vi "Convert Waveform to DDT.vi"() -> ()   [LabVIEW 2011]
doc: "This example shows how to use the Convert to DDT function. Specifically, this example converts the Waveform data type to the Dynamic Data Type, but the Convert to DDT function can also be used to convert 1D or 2D Arrays of doubles and a 1D array of Waveform data. \n\nThe graph plots the multitone wave and the filtered wave. The two signals are combined using the Merge Signals function and have separate Y-axis.\n\nThis example uses the following Express VIs: Convert to DDT and Filter."
uses:
  Instance           2 31Saved   Convert Waveform to DDT .vi
  Instance           3 31Saved   Convert Waveform to DDT .vi
  <vilib>/measure/NI_MAPro.lvlib
panel:
  out "Waveform Graph":dynamicdata(graph)
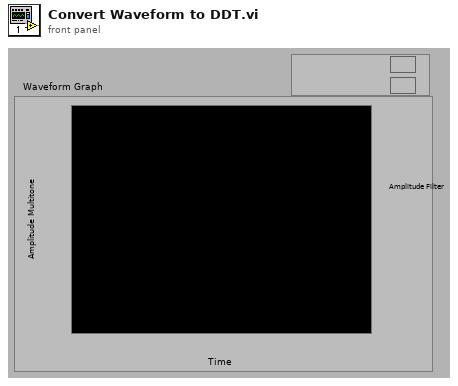
[diagram p1: front panel]
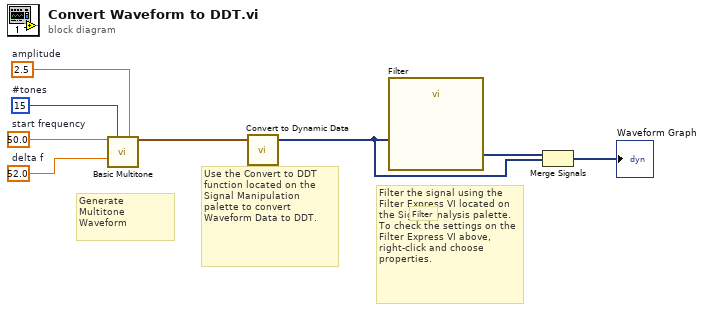
[diagram p0: block diagram]
diagram:
  w5 = 52.0  # delta f
  w6 = 50.0  # start frequency
  w7 = 2.5  # amplitude
  w8 = 15  # #tones
  # "Filter the signal using the Filter Express VI located on the Signal Analysis palette.  To check the settings on the Filter Express VI above, right-click and choose properties."
  # "Use the Convert to DDT function located on the Signal Manipulation palette to convert Waveform Data to DDT."
  # "Filter"
  # "Generate Multitone Waveform"
  n1 = call <vilib>:"Basic Multitone.vi"("start frequency"=w6, "#tones"=w8, "amplitude"=w7, "delta frequency"=w5) -> ("signal out"=w3:waveform(dbl))  [unwired: 6 in, 5 out]
  n2 = call "Convert to Dynamic Data"("Waveform"=w3) -> ("Dynamic Data Type"=w2:dynamicdata)  [unwired: 3 out]
  n3 = call "Filter"("Signal"=w2) -> ("Filtered Signal"=w1:dynamicdata)  [unwired: 3 in, 7 out]
  n4 = Merge Signals "Merge Signals"(w1, w2) -> (→"Waveform Graph":dynamicdata)
